vi "Transfer_Arb_Waveform.vi"(8 "Channel":string="1", 9 "Arbitrary Waveform":dbl[](array[numeric]), 11 "VISA resource name":refnum<visa-resource-name>="USB0::0x0699::0x0347::C036837::INSTR") -> (0 "error out":errorcluster, 3 "VISA resource name out":refnum<visa-resource-name>)   [LabVIEW 2011]
uses:
  <vilib>/Analysis/baseanly.llb/Scale 1D.vi
  <vilib>/Analysis/NI_AALBase.lvlib
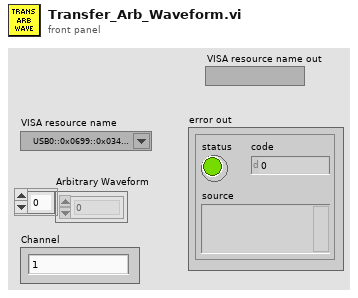
[diagram p1: front panel]
types:
  T1 = enum16{"big-endian, network order", "native, host order", "little-endian"}
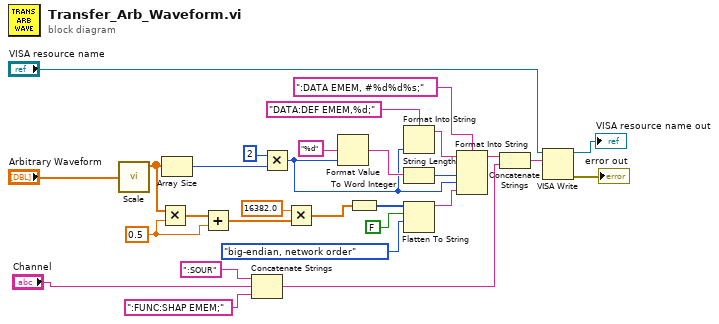
[diagram p0: block diagram]
diagram:
  w22 = 0.5 ("cycles")
  n1 = call-poly <vilib>:"Scale.vi"("X"="Arbitrary Waveform") -> ("Y=(X-offset)/scale"=w19:dbl[])  [unwired: 3 out]
  n2 = Multiply(x=w19, y=w22) -> (x*y=w23:dbl[])
  n3 = Array Size(array=w19) -> (size(s)=w26:i32)
  n4 = Add(x=w23, y=w22) -> (x+y=w21:dbl[])
  n5 = Concatenate Strings(":SOUR" ("string"), "Channel", ":FUNC:SHAP EMEM;" ("write buffer")) -> (w3:string)
  n6 = Multiply(x=2, y=w26) -> (x*y=w12:i32)
  n7 = Multiply(x=16382.0 ("amplitude"), y=w21) -> (x*y=w18:dbl[])
  n8 = Format Value(format string="%d", value (0)=w12) -> (output string=w15:string)  [unwired: 1 in]
  n9 = To Word Integer(number=w18) -> (16bit integer=w27:i16[])
  n10 = Format Into String(format string="DATA:DEF EMEM,%d;", w12) -> (resulting string=w16:string)  [unwired: 2 in, 1 out]
  n11 = String Length(string=w15) -> (length=w13:i32)
  n12 = Flatten To String(anything=w27, prepend array or string size? (T)=FALSE, byte order (0:big-endian, network order)=T1."big-endian, network order") -> (data string=w11:string)  [unwired: 1 in, 2 out]
  n13 = Format Into String(format string=":DATA EMEM, #%d%d%s;", initial string=w16, w13, w12, w11) -> (resulting string=w8:string)  [unwired: 1 in, 1 out]
  n14 = Concatenate Strings(w8, w3) -> (w9:string)
  n15 = VISA Write(VISA resource name="VISA resource name", write buffer=w9) -> (VISA resource name out=→"VISA resource name out":refnum<visa-resource-name>, error out=→"error out":errorcluster)  [unwired: 1 in, 1 out]
